vi "open_test.vi"() -> ()   [LabVIEW 2018]
panel:
  in  "Set mixture":bool
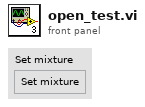
[diagram p1: front panel]
types:
  T1 = enum32{"Invalid", "Standard", "Closed", "Hidden", "Minimized", "Maximized"}
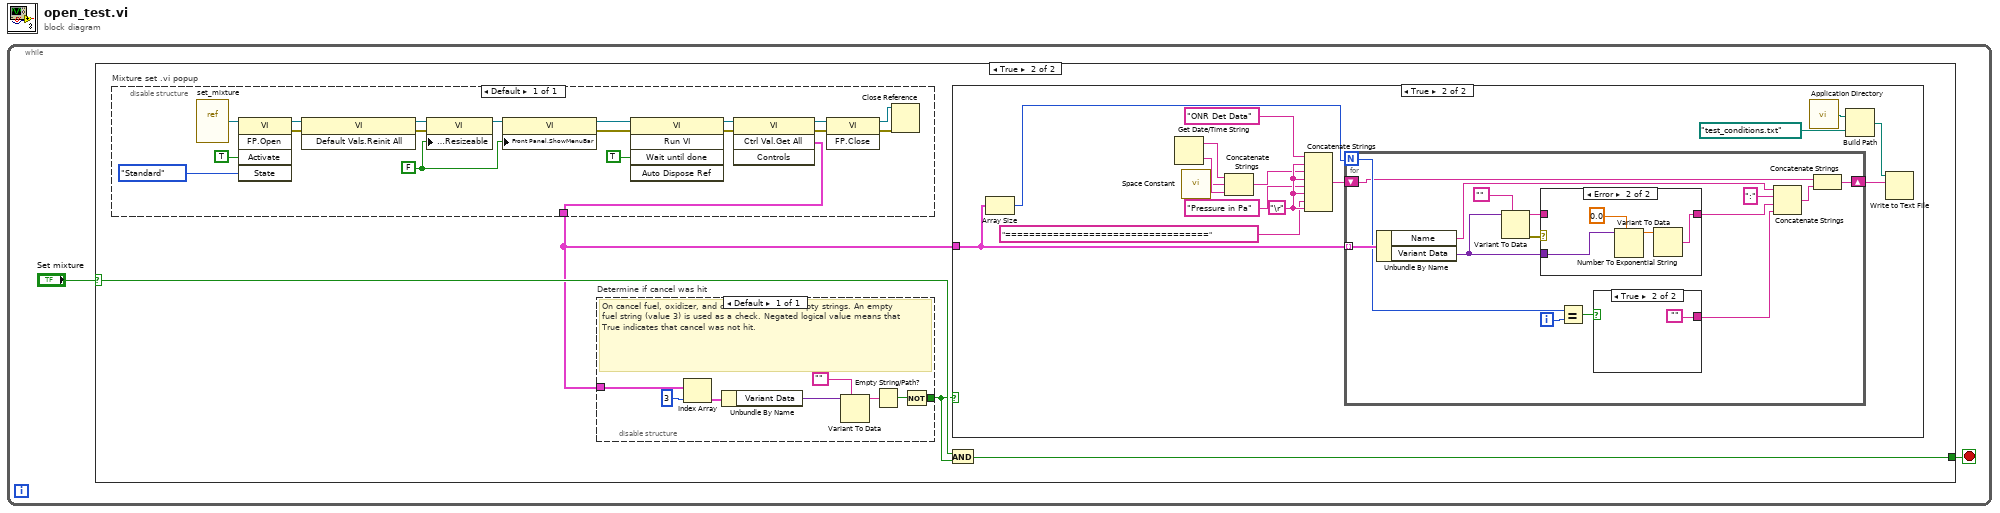
[diagram p0: block diagram]
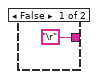
[diagram p5: hidden frame]
diagram:
  n1 = while {
    stop <- w1 stop-if-true
    n2 = case shown="True" "Set mixture" {
      selector: "Set mixture" -> [w3 w7]
      tunnel: [w3 w6] -> w1
      frame False {
      }
      frame True {
        n3 = disable-structure "Mixture set .vi popup" shown="Default" {
          disable-tunnel: [w8] -> w5
          frame Enabled {
            w13 = FALSE ("Front Panel Window:Resizable")
            n4 = vi-ref "set_mixture.vi"() -> (w26:refnum<vi>)
            n5 = invoke class="VI" method="FP.Open"(reference=w26, "Activate"=TRUE ("Activate?"), "State"=T1."Standard") -> (reference out=w16:refnum<vi>, error out=w15:errorcluster)  [unwired: 2 in, 3 out]
            n6 = invoke class="VI" method="Default Vals.Reinit All"(reference=w16, error in=w15) -> (reference out=w12:refnum<vi>, error out=w11:errorcluster)  [unwired: 1 in, 1 out]
            n7 = property class="VI"(reference=w12, error in=w11, "Front Panel.Resizeable"=w13) -> (reference out=w14:refnum<vi>)  [unwired: 1 out]
            n8 = property class="VI"(reference=w14, "Front Panel.ShowMenuBar"=w13) -> (reference out=w10:refnum<vi>, error out=w9:errorcluster)  [unwired: 1 in]
            n9 = invoke class="VI" method="Run VI"(reference=w10, error in=w9, "Wait until done"=TRUE ("Wait Until Done")) -> (reference out=w22:refnum<vi>, error out=w21:errorcluster)  [unwired: 2 in, 3 out]
            n10 = invoke class="VI" method="Ctrl Val.Get All"(reference=w22, error in=w21) -> (reference out=w20:refnum<vi>, error out=w17:errorcluster, "Get All Control Values Variant"=w8:cluster{"Name":string, "Variant Data":variant}[])  [unwired: 2 in, 1 out]
            n11 = invoke class="VI" method="FP.Close"(reference=w20, error in=w17) -> (reference out=w19:refnum<vi>, error out=w18:errorcluster)  [unwired: 1 in, 1 out]
            n12 = Close Reference(reference=w19, error in (no error)=w18) -> ()  [unwired: 1 out]
          }
        }
        n13 = disable-structure "Determine if cancel was hit" shown="Default" {
          disable-tunnel: w5 -> [w67]
          disable-tunnel: [w64] -> w4
          frame Enabled {
            # "On cancel fuel, oxidizer, and diluent will return empty strings. An empty fuel string (value 3) is used as a check. Negated logical value means that True indicates that cancel was not hit."
            n14 = Index Array(array=w67, index=3) -> (element=w69:cluster{"Name":string, "Variant Data":variant})
            n15 = Unbundle By Name(w69) -> ("Variant Data"=w71:variant)
            n16 = Variant To Data(type="", Variant=w71) -> (data=w65:string)  [unwired: 1 in, 1 out]
            n17 = Empty String/Path?(string/path=w65) -> (empty?=w70:bool)
            n18 = Not(x=w70) -> (.not. x?=w64:bool)
          }
        }
        n19 = And(x=w7, y=w4) -> (x .and. y?=w6:bool)
        n20 = case shown="True" w4 {
          tunnel: w5 -> [_ w40]
          frame False {
          }
          frame True {
            w37 = "\r"
            n21 = Array Size(array=w40) -> (size(s)=w41:i32)
            n22 = Get Date/Time String() -> (date string=w33:string, time string=w32:string)  [unwired: 3 in]
            n23 = call <vilib>:"Space Constant.vi"() -> ("String"=w31:string)
            n24 = Concatenate Strings(w33, w31, w32) -> (w34:string)
            n25 = Concatenate Strings("ONR Det Data", w37, w34, w37, "Pressure in Pa", w37, "==================================", w37) -> (w38:string)
            n26 = for {
              N: w41 -> [w52]
              tunnel: w40 -> [w56] mode=indexing
              shift-right: [w46] -> w27
              shift-left: w38 -> [w48]
              i -> [w51]
              n27 = Unbundle By Name(w56) -> ("Name"=w53:string, "Variant Data"=w43:variant)
              n28 = Variant To Data(type="", Variant=w43) -> (data=w44:string, error out=w45:errorcluster)  [unwired: 1 in]
              n29 = case shown="Error" w45 {
                tunnel: [w57 w59] -> w42
                tunnel: w44 -> [w57 _]
                tunnel: w43 -> [_ w61]
                frame No Error {
                }
                frame Error {
                  n30 = Variant To Data(type=0.0, Variant=w61) -> (data=w58:dbl)  [unwired: 1 in, 1 out]
                  n31 = Number To Exponential String(number=w58) -> (E-format string=w59:string)  [unwired: 3 in]
                }
              }
              n32 = Equal?(x=w52, y=w51) -> (x = y?=w50:bool)
              n33 = case shown="True" w50 {
                tunnel: ["\r" ""] -> w49
                frame False {
                }
                frame True {
                }
              }
              n34 = Concatenate Strings(w53, ":", w42, w49) -> (w47:string)
              n35 = Concatenate Strings(w48, w47) -> (w46:string)
            }
            n36 = call <vilib>:"Application Directory.vi"() -> ("Application Directory"=w28:path)
            n37 = Build Path(base path=w28, name or relative path=path "test_conditions.txt" ("file path (use dialog)")) -> (appended path=w30:path)
            n38 = Write to Text File(file (use dialog)=w30, text=w27) -> ()  [unwired: 2 in, 3 out]
          }
        }
      }
    }
  }
